vi "Process.vi"(8 "error in":errorcluster, 11 "Instrument.AFM_DLog in":refnum<class "Instrument.AFM_DLog.lvclass">) -> (0 "error out":errorcluster, 3 "Instrument.AFM_DLog out":refnum<class "Instrument.AFM_DLog.lvclass">)   [LabVIEW 2019, in "Instrument.AFM_DLog.lvclass"]
doc: "---------------------------------------------------------------\nJKI State Machine Objects™\nhttp://jki.net/state-machine-objects/\nCopyright (C) 2005-2015, JKI <info@jki.net>\nALL RIGHTS RESERVED"
uses:
  Instrument.AFM_DLog.lvclass
  <vilib>/JKI/JKI SMO/SMO/SMO.lvclass
  <userlib>/LevyLab/Instrument Framework/Instrument/Instrument.lvclass
  <userlib>/LevyLab/RemoteControl/RemoteControl/Typedefs/Message--Cluster.ctl
  <userlib>/LevyLab/RemoteControl/RemoteControl/RemoteControl.lvclass
  Typedefs/PrivateEvents--AFM_DLog.MessageToProcess.ctl
  <userlib>/LevyLab/Instrument Framework/Instrument Types/SCPI/Instrument.SCPI.lvclass
  <userlib>/LevyLab/Debug/Debug.lvlib
  <userlib>/LevyLab/Instrument Framework/Instrument/API/Instrument.sendMessageToProcess (string).vi
  C:/Program Files (x86)/National Instruments/LabVIEW 2019/vi.lib/JKI/JKI SMO/SMO/SMO.lvclass
  C:/Program Files (x86)/National Instruments/LabVIEW 2019/user.lib/LevyLab/Instrument Framework/Instrument/Instrument.lvclass
panel:
  out "Status":string
  out "State History":string
  # "Instrument.Framework-Template"
  # "Framework-Template"
  # "For instructions on how to use the JKI State Machine Objects, examples and video tutorials, visit:\nhttp://jki.net/state-machine-objects/\n\nJKI State Machine Objects™\nhttp://jki.net/state-machine-objects/\nCopyright (C) 2005-2015, JKI <info@jki.net>\nALL RIGHTS RESERVED"
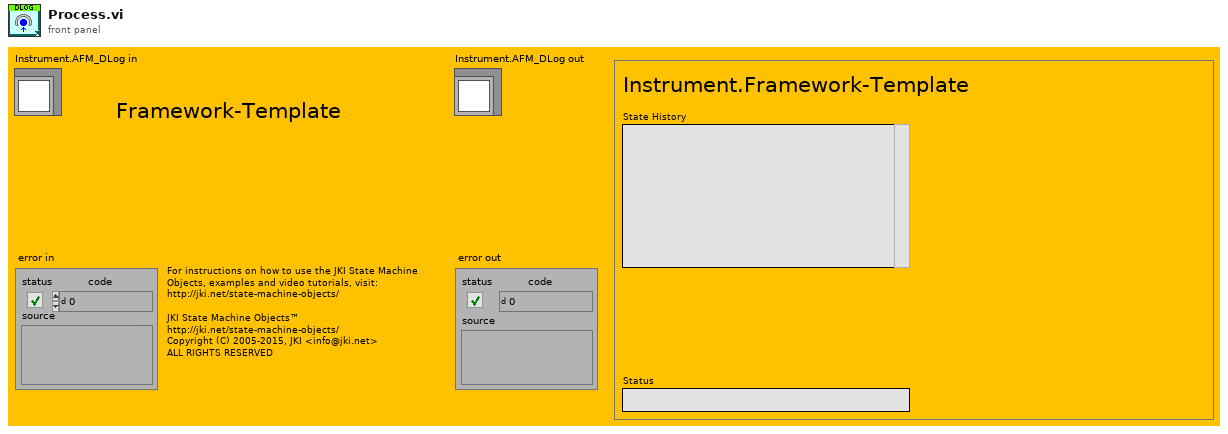
[diagram p1: front panel]
types:
  T1 = enum32{"invalid app kind", "Development System", "Run Time System", "Student Edition", "Embedded LabVIEW", "Evaluation", "Custom"}
  T2 = enum32{"Invalid", "Standard", "Closed", "Hidden", "Minimized", "Maximized"}
  T3 = typedef "RemoteControl.lvlib/RemoteControl.lvclass/Message--Cluster.ctl" = cluster{"Command":string, "Data":variant, "ID":string}
  T4 = typedef "Instrument.AFM_DLog.lvclass/PrivateEvents--AFM_DLog.MessageToProcess.ctl" = cluster{"Message":T3}
  T5 = cluster{"Core":cluster{"Current VI Reference":refnum<vi>, "Close Panel on Exit?":bool, "Last Error":cluster{"error":errorcluster, "previous state":string, "remaining states":string}, "Shutdown?":bool}, "SelfRef":refnum<class "Instrument.AFM_DLog.lvclass">, "HAL":refnum<class "HAL.lvclass">, "Running Step":i32, "sequence":string[], "MessageToProcess":T4, "UI Behavior":string, "wait":u32}
  T6 = cluster{"Current VI Reference":refnum<vi>, "Close Panel on Exit?":bool, "Last Error":cluster{"error":errorcluster, "previous state":string, "remaining states":string}, "Shutdown?":bool}
  T7 = typedef "Debug.lvlib/Attribute.Debug.lvclass/DebugBehavior.ctl" = enum16{"Normal", "Debug"}
  T8 = typedef "smo.lvlib/SMO.lvclass/Protected Events.ctl" = cluster{"StopProcesses":refnum<user-event>, "AbortProcesses":refnum<user-event>, "Config Changed":refnum<user-event>, "Dependency":refnum<user-event>}
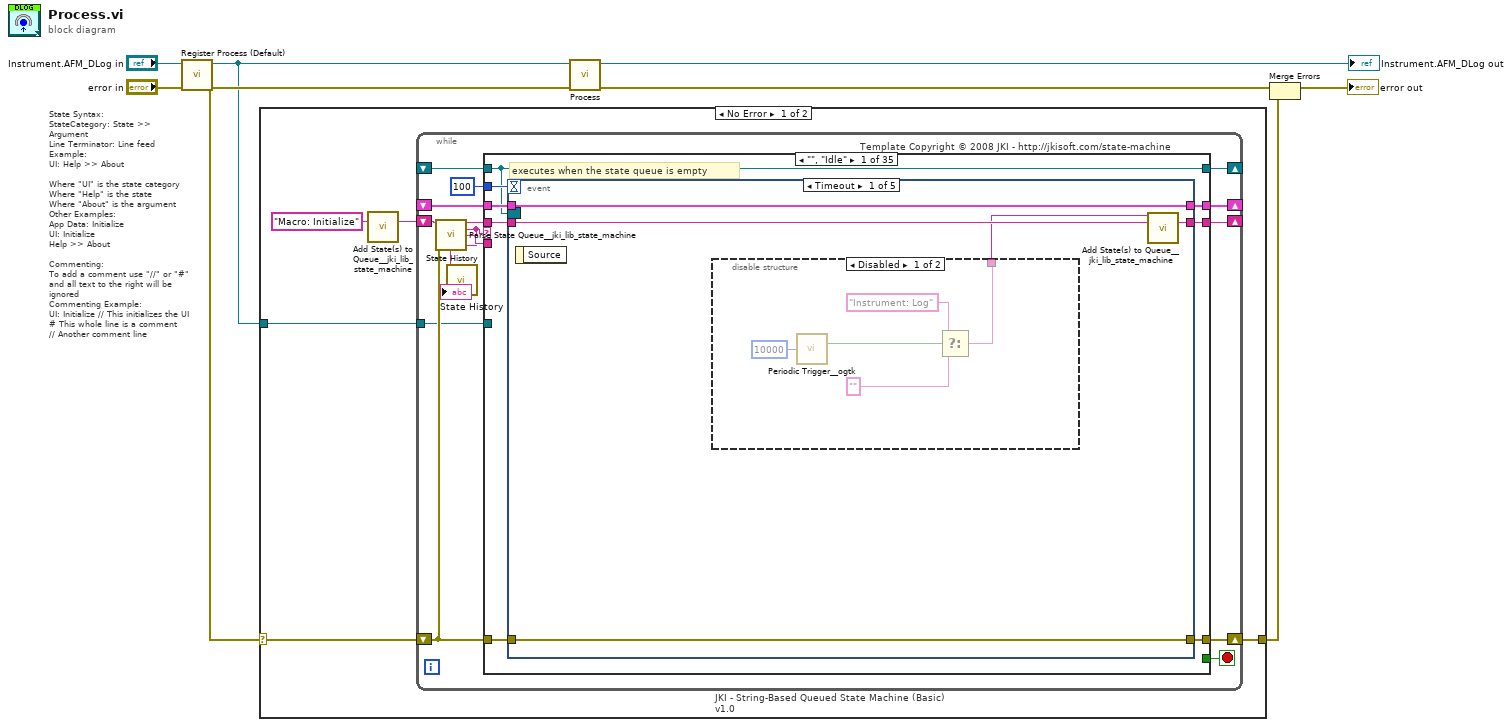
[diagram p0: block diagram]
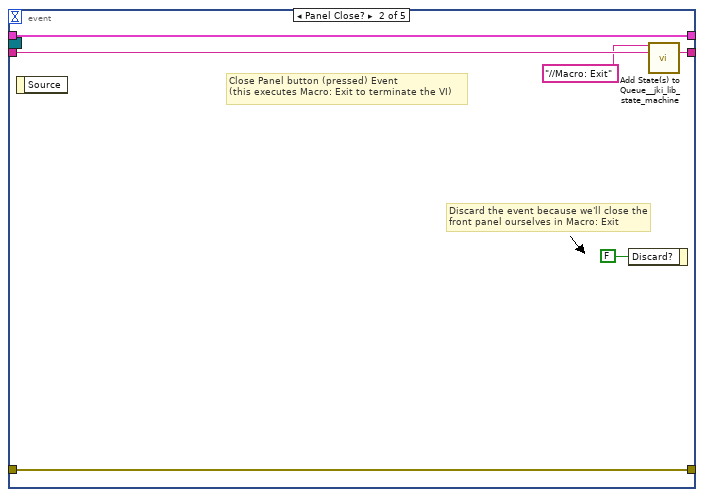
[diagram p3: hidden frame]
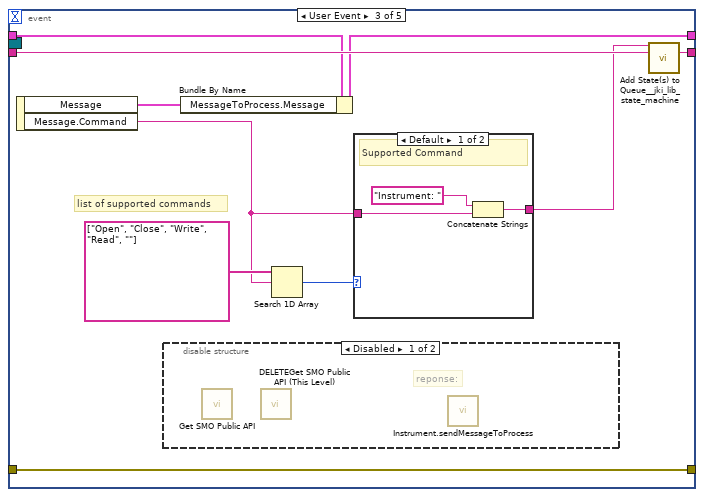
[diagram p4: hidden frame]
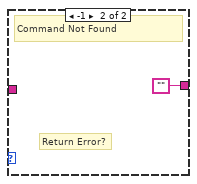
[diagram p6: hidden frame]
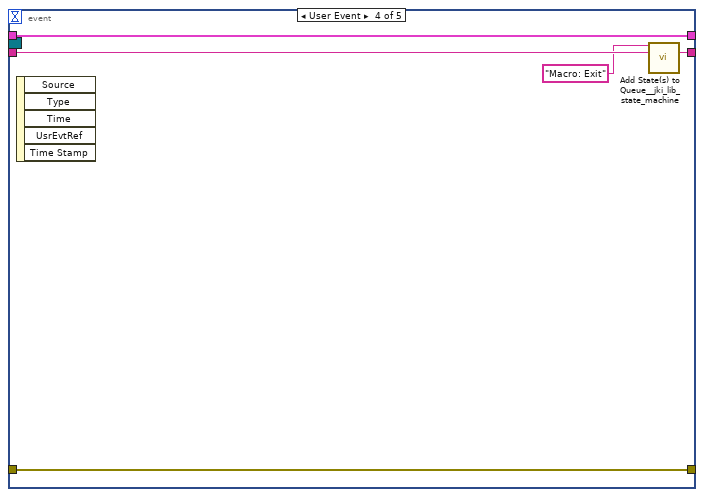
[diagram p7: hidden frame]
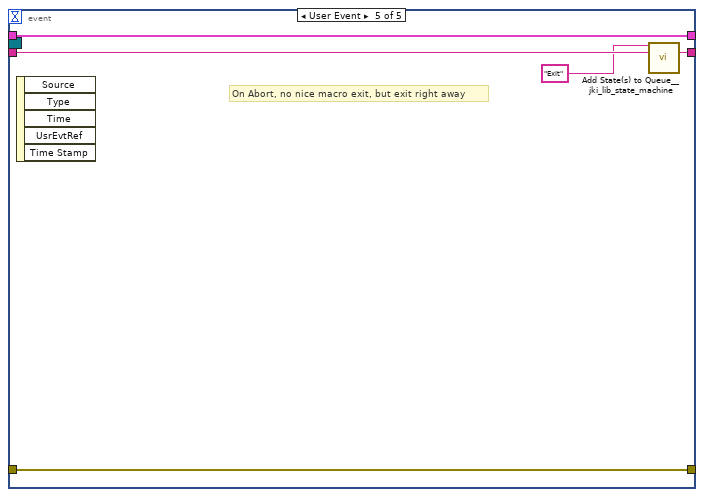
[diagram p8: hidden frame]
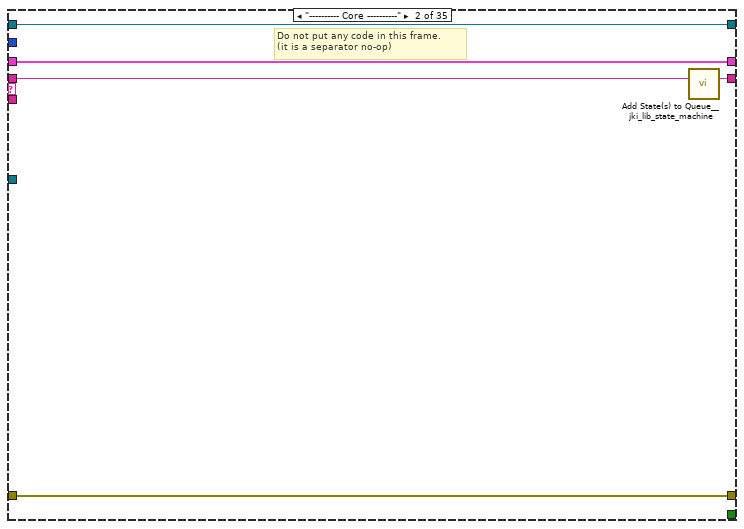
[diagram p9: hidden frame]
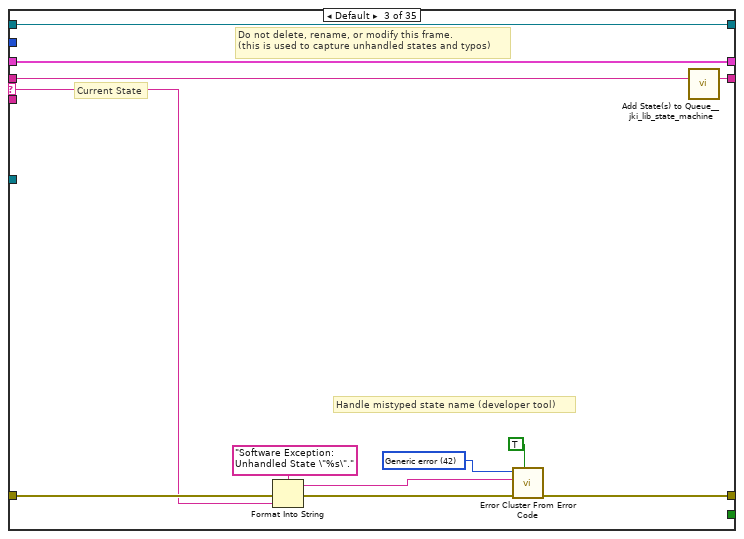
[diagram p10: hidden frame]
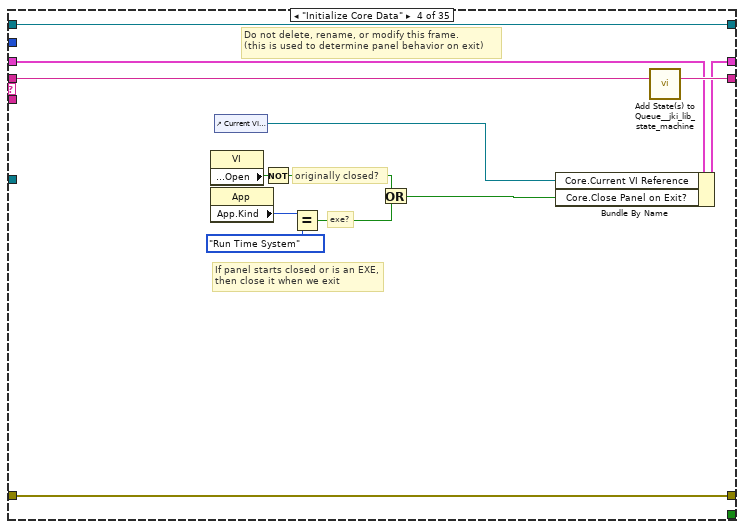
[diagram p11: hidden frame]
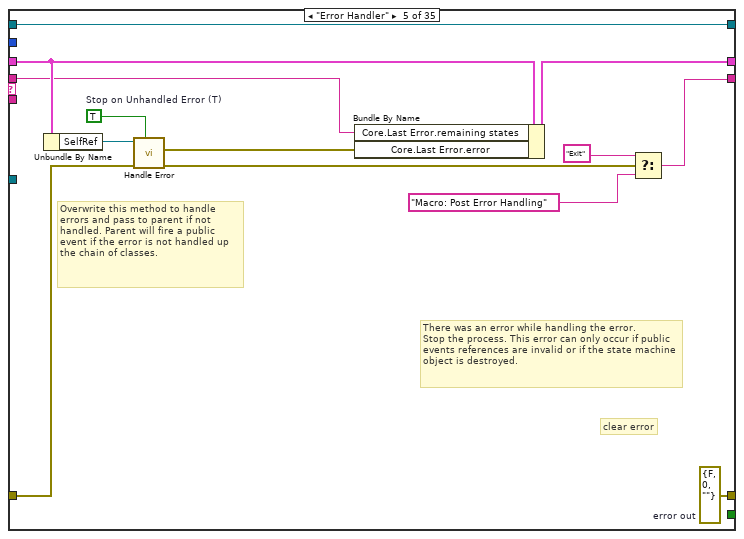
[diagram p12: hidden frame]
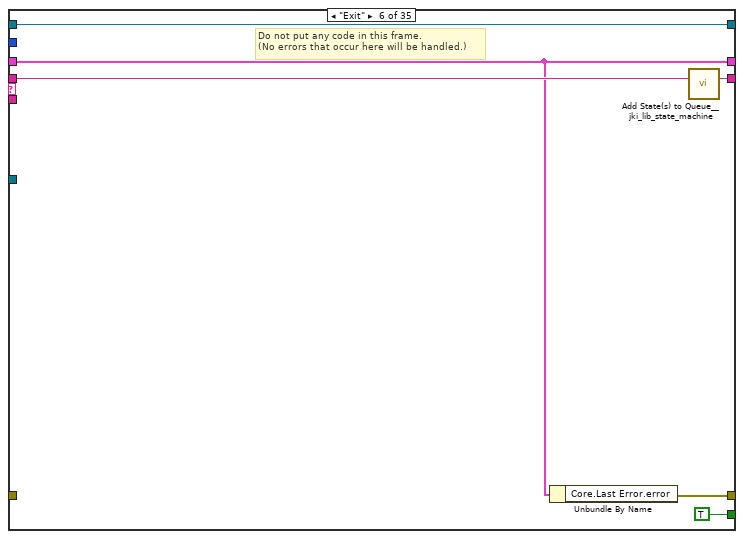
[diagram p13: hidden frame]
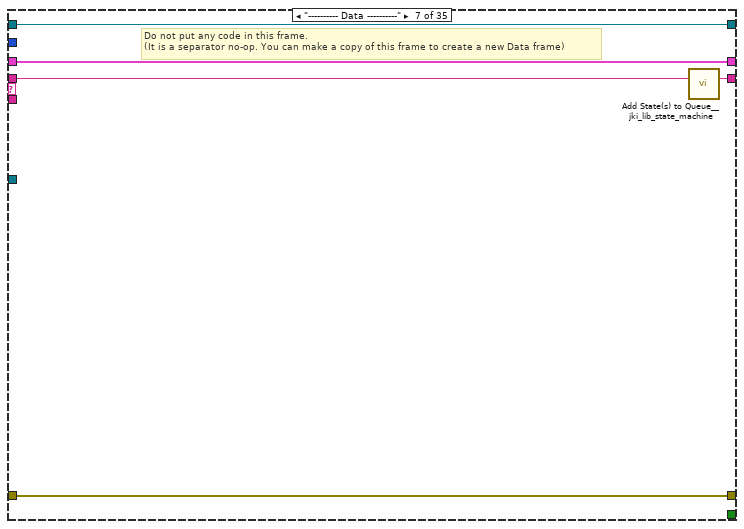
[diagram p14: hidden frame]
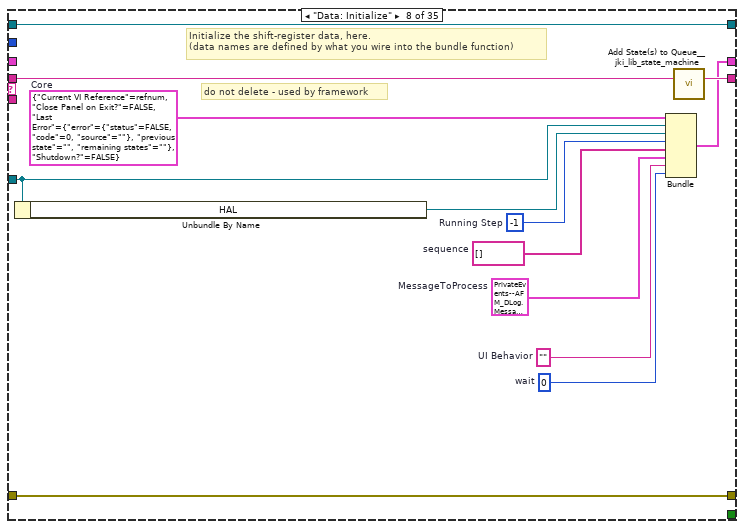
[diagram p15: hidden frame]
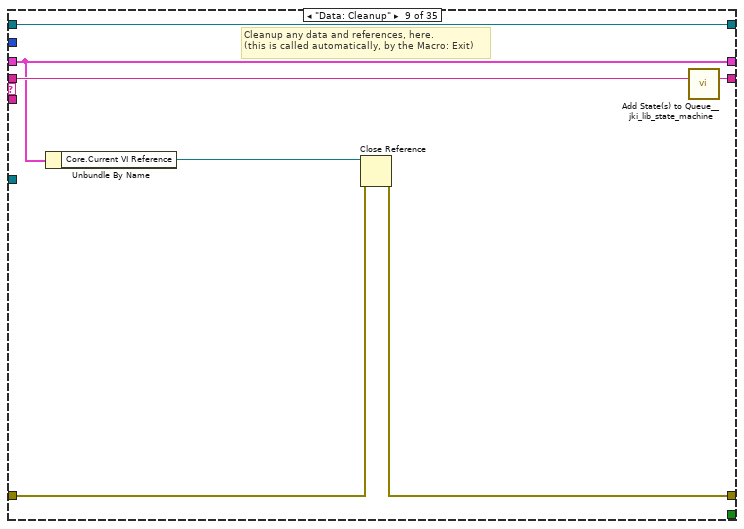
[diagram p16: hidden frame]
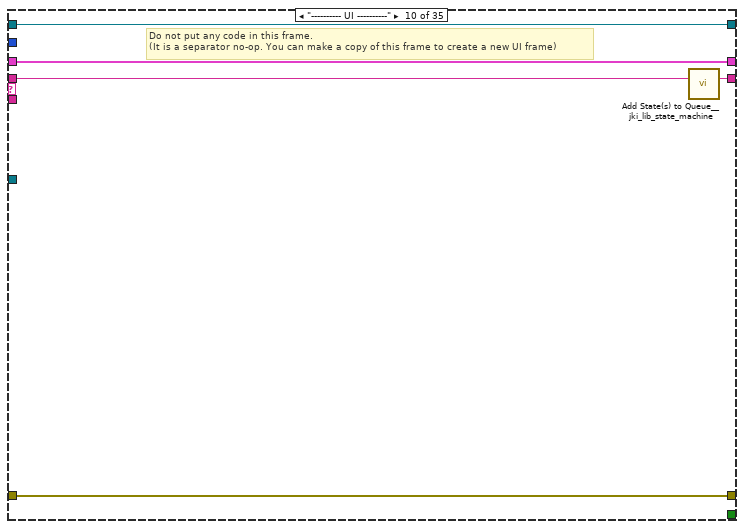
[diagram p17: hidden frame]
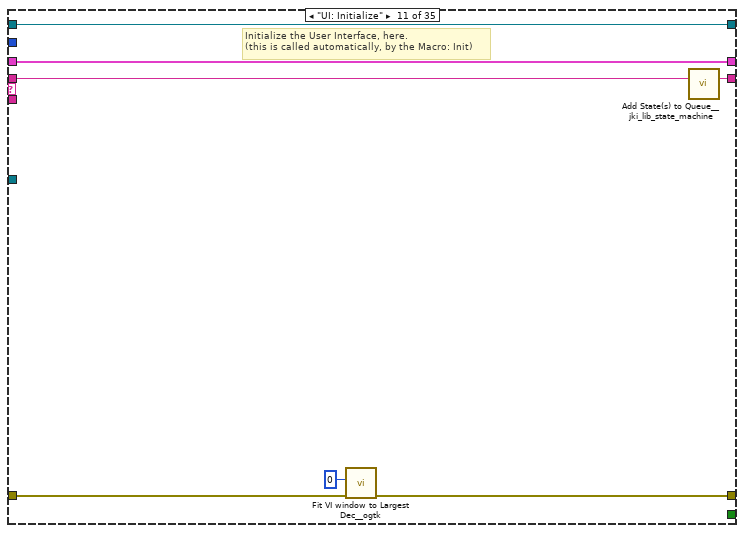
[diagram p18: hidden frame]
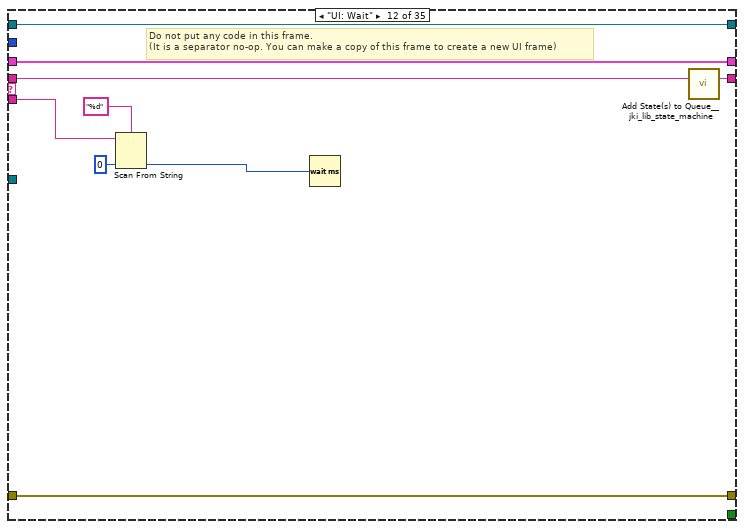
[diagram p19: hidden frame]
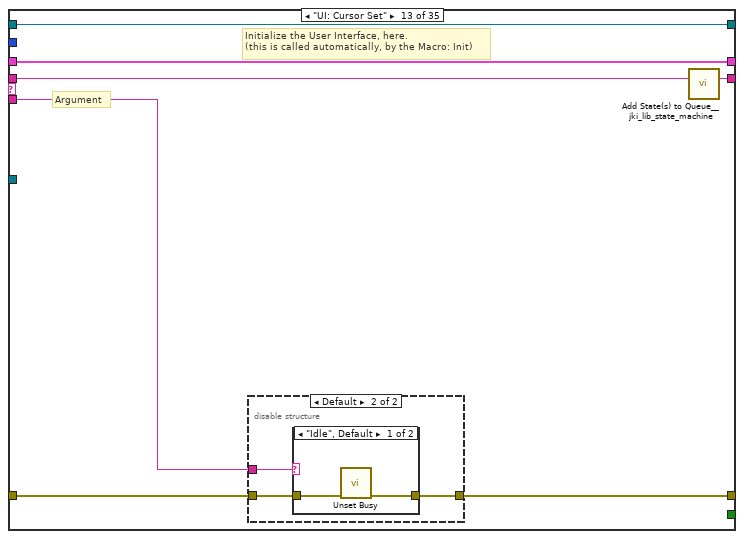
[diagram p20: hidden frame]
diagram:
  # "State Syntax:\nStateCategory: State >> Argument\nLine Terminator: Line feed\nExample:\nUI: Help >> About\n\nWhere \"UI\" is the state category\nWhere \"Help\" is the state\nWhere \"About\" is the argument\nOther Examples:\nApp Data: Initialize\nUI: Initialize\nHelp >> About\n\nCommenting:\nTo add a comment use \"//\" or \"#\" and all text to the right will be ignored\nCommenting Example:\nUI: Initialize // This initializes the UI\n# This whole line is a comment\n// Another comment line"
  n1 = call <vilib>:"Register Process (Default).vi"("error in (no error)"="error in", "SMO"="Instrument.AFM_DLog in") -> ("error out"=w5:errorcluster, "SelfRef"=w4:refnum<class "Instrument.AFM_DLog.lvclass">)  [unwired: 8 in]
  n2 = case shown="No Error" w5 {
    selector: w5 -> [w10 w455]
    tunnel: w4 -> [w11 _]
    tunnel: [w9 w455] -> w1
    frame No Error {
      n3 = call <vilib>:"Add State(s) to Queue__jki_lib_state_machine.vi"("State(s) in (\"\")"="Macro: Initialize") -> ("States Out"=w13:string)  [unwired: 14 in]
      n4 = while "JKI - String-Based Queued State Machine (Basic) v1.0" {
        shift-right: [w22] -> _
        shift-left: _ -> [w21]
        shift-right: [w25] -> w9
        shift-left: w10 -> [w19]
        shift-right: [w24] -> _
        shift-left: w13 -> [w26]
        tunnel: w11 -> [w18]
        shift-right: [w17] -> _
        shift-left: _ -> [w16]
        stop <- w23 stop-if-true
        # "Template Copyright © 2008 JKI - http://jkisoft.com/state-machine"
        n5 = call <vilib>:"Parse State Queue__jki_lib_state_machine.vi"("State Queue"=w26, "Error In (no error)"=w19) -> ("Remaining States"=w28:string, "Current State"=w15:string, "Arguments"=w27:string)  [unwired: 11 in]
        n6 = call <userlib>:"State History.vi"("Current State"=w15) -> ("History"=→"State History":string)  [unwired: 10 in]
        n7 = case shown="\"\", \"Idle\"" w15 {
          selector: w15 -> [_ _ w83 _ _ _ _ _ _ _ _ _ _ _ _ _ _ _ _ _ _ _ _ _ _ _ _ _ _ _ _ _ _ _ _]
          tunnel: w28 -> [w36 w81 w87 w106 w111 w125 w130 w143 w150 w155 w162 w171 w178 w194 w226 w235 w247 w268 w283 w305 w310 w321 w326 w339 w345 w353 w362 w371 w381 w390 w405 w424 w429 w435 w454]
          tunnel: w27 -> [_ _ _ _ _ _ _ _ _ _ _ w163 w172 w188 _ _ _ _ _ _ _ _ _ _ _ _ _ _ _ _ _ _ _ w430 w438]
          tunnel: w21 -> [w34 w78 w85 w97 w115 w121 w127 _ w145 w152 w160 w168 w176 w190 w223 w232 w237 w258 w272 w290 w307 w318 w323 w332 w343 w348 w358 w367 w377 w386 w401 w420 w425 w431 w444]
          tunnel: [w33 w79 w89 w103 w116 w120 w128 w133 w146 w153 w157 w169 w173 w191 w224 w227 w245 w266 w271 w293 w308 w312 w324 w335 w341 w350 w354 w366 w376 w385 w395 w418 w426 w432 w446] -> w25
          tunnel: w19 -> [w32 w79 w88 w103 w117 _ w128 w133 w147 w153 w156 w169 w174 w192 w224 w227 w245 w266 w270 w293 w308 w313 w324 w329 w341 w350 w357 w365 w375 w384 w399 w416 w426 w432 w440]
          tunnel: [w35 w80 w86 w105 w107 w124 w129 w142 w149 w154 w161 w170 w177 w193 w225 w234 w246 w267 w282 w304 w309 w320 w325 w338 w344 w352 w361 w370 w380 w389 w404 w423 w428 w434 w453] -> w24
          tunnel: [_ _ _ _ _ TRUE _ _ _ _ _ _ _ _ _ _ _ _ _ _ _ _ _ _ _ _ _ _ _ _ _ _ _ _ _] -> w23
          tunnel: [w31 w78 w85 w104 w114 w121 w127 w141 w145 w152 w160 w168 w176 w190 w223 w232 w238 w259 w273 w291 w307 w318 w323 w332 w343 w349 w359 w368 w378 w387 w402 w421 w425 w431 w443] -> w22
          tunnel: 100 ("Timeout") -> [w30 _ _ _ _ _ _ _ _ _ _ _ _ _ _ _ _ _ _ _ _ _ _ _ _ _ _ _ _ _ _ _ _ _ _]
          tunnel: w18 -> [_ _ _ _ _ _ _ w134 _ _ _ _ _ _ _ _ _ _ _ _ _ _ _ _ _ _ _ _ _ _ _ _ _ _ _]
          tunnel: [w29 w77 w82 w94 w119 w122 w126 w140 w144 w151 w159 w167 w175 w187 w222 w233 w244 w265 w281 w299 w306 w319 w322 w337 w342 w351 w360 w369 w379 w388 w403 w422 w427 w433 w452] -> w17
          tunnel: w16 -> [w29 w77 w82 w94 w119 w122 w126 w140 w144 w151 w159 w167 w175 w187 w222 w233 w244 w265 w281 w299 w306 w319 w322 _ w342 w351 w360 w369 w379 w388 w403 w422 w427 w433 w452]
          frame "", "Idle" {
            # "executes when the state queue is empty"
            n8 = event shown="[0] Timeout" {
              selector: w29 -> [_ _ _ _ _]
              dyn-events: _ -> [_ _ _ _ _]
              timeout: w30 -> [_ _ _ _ _]
              tunnel: w36 -> [w41 w52 w62 w71 w76]
              tunnel: [w40 w51 w61 w70 w75] -> w35
              tunnel: w34 -> [w38 w49 w54 w68 w73]
              tunnel: [w39 w50 w60 w69 w74] -> w33
              tunnel: w32 -> [w39 w50 w60 w69 w74]
              tunnel: [w38 w49 w55 w68 w73] -> w31
              event Timeout {
                n9 = event-data() -> ()  [unwired: 1 in, 1 out]
                n10 = disable-structure shown="Disabled" {
                  disable-tunnel: [w45 _] -> w37
                  frame Disabled {
                    n11 = call <userlib>:"Periodic Trigger__ogtk.vi"("time (ms)"=u32 10000) -> ("Triggered"=w44:bool)  [unwired: 12 in, 2 out]
                    n12 = Select(t="Instrument: Log", s=w44, f="") -> (s? t:f=w45:string)
                  }
                  frame Enabled {
                  }
                }
                n13 = call <vilib>:"Add State(s) to Queue__jki_lib_state_machine.vi"("State(s) in Front (\"\")"=w37, "State(s) in (\"\")"=w41) -> ("States Out"=w40:string)  [unwired: 13 in]
              }
              event Panel Close? {
                # "Discard the event because we'll close the front panel ourselves in Macro: Exit"
                # "Close Panel button (pressed) Event\n(this executes Macro: Exit to terminate the VI)"
                n14 = event-data() -> ()  [unwired: 1 in, 1 out]
                n15 = event-data("Discard?"=FALSE) -> ()  [unwired: 1 in, 1 out]
                n16 = call <vilib>:"Add State(s) to Queue__jki_lib_state_machine.vi"("State(s) in Front (\"\")"="//Macro: Exit", "State(s) in (\"\")"=w52) -> ("States Out"=w51:string)  [unwired: 13 in]
              }
              event User Event {
                # "list of supported commands"
                n17 = event-data() -> ("Message"=w53:T3, "Message.Command"=w56:string)  [unwired: 1 in]
                n18 = disable-structure shown="Disabled" {
                  frame Disabled {
                    # "reponse:"
                    n19 = call-dynamic "Get SMO Public API.vi"() -> ()  [unwired: 9 in, 3 out]
                    n20 = call-dynamic "DELETEGet SMO Public API (This Level).vi"() -> ()  [unwired: 9 in, 3 out]
                    n21 = call-poly <userlib>:"Instrument.sendMessageToProcess.vi"() -> ()  [unwired: 10 in, 2 out]
                  }
                  frame Enabled {
                  }
                }
                n22 = Bundle By Name(cluster=w54, "MessageToProcess.Message"=w53) -> (w55:T5)
                n23 = Search 1D Array(1D array=string[] ["Open", "Close", "Write", "Read", ""], element=w56) -> (index of element=w59:i32)  [unwired: 1 in]
                n24 = case shown="Default" w59 {
                  tunnel: [w65 "" ("Empty String Constant")] -> w57
                  tunnel: w56 -> [w64 _]
                  frame Default {
                    # "Supported Command"
                    n25 = Concatenate Strings("Instrument: ", w64) -> (w65:string)
                  }
                  frame -1 {
                    # "Return Error?"
                    # "Command Not Found"
                  }
                }
                n26 = call <vilib>:"Add State(s) to Queue__jki_lib_state_machine.vi"("State(s) in Front (\"\")"=w57, "State(s) in (\"\")"=w62) -> ("States Out"=w61:string)  [unwired: 13 in]
              }
              event User Event {
                n27 = event-data() -> ()  [unwired: 1 in, 5 out]
                n28 = call <vilib>:"Add State(s) to Queue__jki_lib_state_machine.vi"("State(s) in Front (\"\")"="Macro: Exit", "State(s) in (\"\")"=w71) -> ("States Out"=w70:string)  [unwired: 13 in]
              }
              event User Event {
                # "On Abort, no nice macro exit, but exit right away"
                n29 = event-data() -> ()  [unwired: 1 in, 5 out]
                n30 = call <vilib>:"Add State(s) to Queue__jki_lib_state_machine.vi"("State(s) in Front (\"\")"="Exit", "State(s) in (\"\")"=w76) -> ("States Out"=w75:string)  [unwired: 13 in]
              }
            }
          }
          frame "---------- Core ----------" {
            # "Do not put any code in this frame.\n(it is a separator no-op)"
            n31 = call <vilib>:"Add State(s) to Queue__jki_lib_state_machine.vi"("State(s) in (\"\")"=w81) -> ("States Out"=w80:string)  [unwired: 14 in]
          }
          frame Default {
            w92 = 42 items=["No error", "Argument error", "Memory is full", "Out of zone", "End of file", "File already open", "Generic file I/O error", "File not found", "File permission error", "Disk is full", "Duplicate path", "Too many files open", "System feature not enabled", "Resource file not found", "Cannot add resource", "Resource not found", "Image not found", "Image memory error", "Pen does not exist", "Config type invalid", "Config token not found", "Config parse error", "Config memory error", "Bad external code format", "Bad external code offset", "External code not present", "Null window", "Destroy window error", "Null menu", "Print aborted", "Bad print record", "Print driver error", "Windows error during printing", "Memory error during printing", "Print dialog error", "Generic print error", "Invalid device refnum", "Device not found", "Device parameter error", "Device unit error", "Cannot open device", "Device call aborted", "Generic error", "Cancelled by user", "Object ID too low", "Object ID too high", "Object not in heap", "Unknown heap", "Unknown object (invalid DefProc)", "Unknown object (DefProc not in table)", "Message out of range", "Invalid (null) method", "Unknown message", "Manager call not supported", "Bad address", "Network operation in progress", "Network operation timed out", "Connection is busy", "Network attribute not supported", "Network error", "Address in use", "System out of memory", "Connection aborted", "Connection refused", "Not connected", "Already connected", "Connection closed", "Initialization error (interapplication manager)", "Bad occurrence", "Wait on unbound occurrence handler", "Occurrence queue overflow", "Datalog type conflict", "Unused", "Unrecognized type (interapplication manager)", "Memory corrupt", "Failed to make temporary DLL", "Old CIN version", "Drag socket not found", "Failed to load drop-object", "Failed to register OLE object", "Failed to release OLE object", "Format specifier type mismatch", "Unknown format specifier", "Too few format specifiers", "Too many format specifiers", "Scan failed", "Newer CIN version", "Error converting to variant", "Runtime menu error", "Password tampered", "Variant attribute not found", "Incompatible variant data type", "Event data is not available", "Event Store is not present", "Occurrence is not found", "Event Queue is not created", "Event info is not available", "Refnum passed is NULL", "Error retrieving Class GUID", "Error retrieving CoClass GUID", "Error retrieving TypeLib GUID.", "Bad built application magic bytes.", "Specific driver is different from the specific driver associated with the Logical Name.", "There is no session opened to the class driver.", "Max Error", "MAX - Error with config objects", "MAX - Error loading configuration", "MAX - Group not supported"]
            # "Current State"
            # "Do not delete, rename, or modify this frame.\n(this is used to capture unhandled states and typos)"
            # "Handle mistyped state name (developer tool)"
            n32 = Format Into String(format string="Software Exception: Unhandled State \"%s\"." ("message"), error in=w88, w83) -> (resulting string=w91:string, error out=w90:errorcluster)  [unwired: 1 in]
            n33 = call <vilib>:"Error Cluster From Error Code.vi"("show call chain? (False)"=TRUE, "error in (no error)"=w90, "error message (\"\")"=w91, "error code (0)"=w92) -> ("error out"=w89:errorcluster)  [unwired: 5 in]
            n34 = call <vilib>:"Add State(s) to Queue__jki_lib_state_machine.vi"("State(s) in (\"\")"=w87) -> ("States Out"=w86:string)  [unwired: 14 in]
          }
          frame "Initialize Core Data" {
            # "Do not delete, rename, or modify this frame.\n(this is used to determine panel behavior on exit)"
            # "originally closed?"
            # "exe?"
            # "If panel starts closed or is an EXE, then close it when we exit"
            n35 = property class="VI"() -> ("Front Panel.Open"=w102:bool)  [unwired: 2 in, 2 out]
            n36 = property class="App"() -> ("App.Kind"=w101:T1)  [unwired: 2 in, 2 out]
            n37 = control-ref of="Current VI Reference"() -> (w95:refnum<vi>)
            n38 = Not(x=w102) -> (.not. x?=w99:bool)
            n39 = Equal?(x=w101, y=T1."Run Time System" ("Application:Kind")) -> (x = y?=w98:bool)
            n40 = Or(x=w99, y=w98) -> (x .or. y?=w96:bool)
            n41 = Bundle By Name(cluster=w97, "Core.Current VI Reference"=w95, "Core.Close Panel on Exit?"=w96) -> (w104:T5)
            n42 = call <vilib>:"Add State(s) to Queue__jki_lib_state_machine.vi"("State(s) in (\"\")"=w106) -> ("States Out"=w105:string)  [unwired: 14 in]
          }
          frame "Error Handler" {
            w112 = TRUE  # Stop on Unhandled Error (T)
            w116 = errorcluster {"status"=FALSE, "code"=0, "source"=""}  # error out
            # "clear error"
            # "There was an error while handling the error.\nStop the process. This error can only occur if public events references are invalid or if the state machine object is destroyed."
            # "Overwrite this method to handle errors and pass to parent if not handled. Parent will fire a public event if the error is not handled up the chain of classes."
            n43 = Unbundle By Name(w115) -> ("SelfRef"=w118:refnum<class "Instrument.AFM_DLog.lvclass">)
            n44 = call-dynamic "Handle Error.vi"("Stop on Unhandled Error (T)"=w112, "error in"=w117, "SMO"=w118) -> ("handling error"=w108:errorcluster, "Unhandled error"=w113:errorcluster)  [unwired: 6 in, 1 out]
            n45 = Bundle By Name(cluster=w115, "Core.Last Error.remaining states"=w111, "Core.Last Error.error"=w113) -> (w114:T5)
            n46 = Select(t="Exit", s=w108, f="Macro: Post Error Handling") -> (s? t:f=w107:string)
          }
          frame "Exit" {
            # "Do not put any code in this frame.\n(No errors that occur here will be handled.)"
            n47 = Unbundle By Name(w121) -> ("Core.Last Error.error"=w120:errorcluster)
            n48 = call <vilib>:"Add State(s) to Queue__jki_lib_state_machine.vi"("State(s) in (\"\")"=w125) -> ("States Out"=w124:string)  [unwired: 14 in]
          }
          frame "---------- Data ----------" {
            # "Do not put any code in this frame.\n(It is a separator no-op. You can make a copy of this frame to create a new Data frame)"
            n49 = call <vilib>:"Add State(s) to Queue__jki_lib_state_machine.vi"("State(s) in (\"\")"=w130) -> ("States Out"=w129:string)  [unwired: 14 in]
          }
          frame "Data: Initialize" {
            w131 = u32 0  # wait
            w132 = ""  # UI Behavior
            w136 = T4 {"Message"={"Command"="", "Data"=variant(string ""), "ID"=""}}  # MessageToProcess
            w137 = string[] []  # sequence
            w138 = -1  # Running Step
            w139 = T6 {"Current VI Reference"=refnum, "Close Panel on Exit?"=FALSE, "Last Error"={"error"={"status"=FALSE, "code"=0, "source"=""}, "previous state"="", "remaining states"=""}, "Shutdown?"=FALSE}  # Core
            # "do not delete - used by framework"
            # "Initialize the shift-register data, here.\n(data names are defined by what you wire into the bundle function)"
            n50 = Unbundle By Name(w134) -> ("HAL"=w135:refnum<class "HAL.lvclass">)
            n51 = Bundle("Core"=w139, "SelfRef"=w134, "HAL"=w135, "Running Step"=w138, "sequence"=w137, "MessageToProcess"=w136, "UI Behavior"=w132, "wait"=w131) -> (w141:T5)  [unwired: 1 in]
            n52 = call <vilib>:"Add State(s) to Queue__jki_lib_state_machine.vi"("State(s) in (\"\")"=w143) -> ("States Out"=w142:string)  [unwired: 14 in]
          }
          frame "Data: Cleanup" {
            # "Cleanup any data and references, here.\n(this is called automatically, by the Macro: Exit)"
            n53 = Unbundle By Name(w145) -> ("Core.Current VI Reference"=w148:refnum<vi>)
            n54 = Close Reference(reference=w148, error in (no error)=w147) -> (error out=w146:errorcluster)
            n55 = call <vilib>:"Add State(s) to Queue__jki_lib_state_machine.vi"("State(s) in (\"\")"=w150) -> ("States Out"=w149:string)  [unwired: 14 in]
          }
          frame "---------- UI ----------" {
            # "Do not put any code in this frame.\n(It is a separator no-op. You can make a copy of this frame to create a new UI frame)"
            n56 = call <vilib>:"Add State(s) to Queue__jki_lib_state_machine.vi"("State(s) in (\"\")"=w155) -> ("States Out"=w154:string)  [unwired: 14 in]
          }
          frame "UI: Initialize" {
            # "Initialize the User Interface, here.\n(this is called automatically, by the Macro: Init)"
            n57 = call <userlib>:"Fit VI window to Largest Dec__ogtk.vi"("error in (no error)"=w156, "border spacing (2 px)"=0) -> ("error out"=w157:errorcluster)  [unwired: 4 in, 1 out]
            n58 = call <vilib>:"Add State(s) to Queue__jki_lib_state_machine.vi"("State(s) in (\"\")"=w162) -> ("States Out"=w161:string)  [unwired: 14 in]
          }
          frame "UI: Wait" {
            # "Do not put any code in this frame.\n(It is a separator no-op. You can make a copy of this frame to create a new UI frame)"
            n59 = Scan From String(format string="%d", input string=w163, default 1=u32 0 ("default value 1")) -> (output 1=w164:u32)  [unwired: 2 in, 3 out]
            n60 = Wait (ms)(milliseconds to wait=w164) -> ()  [unwired: 1 out]
            n61 = call <vilib>:"Add State(s) to Queue__jki_lib_state_machine.vi"("State(s) in (\"\")"=w171) -> ("States Out"=w170:string)  [unwired: 14 in]
          }
          frame "UI: Cursor Set" {
            # "Argument"
            # "Initialize the User Interface, here.\n(this is called automatically, by the Macro: Init)"
            n62 = disable-structure shown="Default" {
              disable-tunnel: w174 -> [w179 w182]
              disable-tunnel: [w179 w181] -> w173
              disable-tunnel: w172 -> [_ w180]
              frame condition #0 {
              }
              frame condition #1 (active) {
                n63 = case shown="\"Idle\", Default" w180 {
                  tunnel: w182 -> [w184 w186]
                  tunnel: [w183 w185] -> w181
                  frame "Idle", Default {
                    n64 = call <vilib>:"Unset Busy.vi"("error in (no error)"=w184) -> ("error out"=w183:errorcluster)  [unwired: 10 in]
                  }
                  frame "Busy" {
                    n65 = call <vilib>:"Set Busy.vi"("error in (no error)"=w186) -> ("error out"=w185:errorcluster)  [unwired: 9 in, 1 out]
                  }
                }
              }
            }
            n66 = call <vilib>:"Add State(s) to Queue__jki_lib_state_machine.vi"("State(s) in (\"\")"=w178) -> ("States Out"=w177:string)  [unwired: 14 in]
          }
          frame "UI: Front Panel State" {
            # "Argument"
            # "Set Front Panel Open or Closed\n(Usage: \"UI: Front Panel State >> Open|Close\")"
            n67 = Unbundle By Name(w190) -> ("Core.Current VI Reference"=w189:refnum<vi>)
            n68 = disable-structure shown="TARGET_TYPE==RT" {
              disable-tunnel: w192 -> [w198 w221]
              disable-tunnel: [w197 w221] -> w191
              disable-tunnel: w189 -> [w196 _]
              disable-tunnel: w188 -> [w195 _]
              frame condition #0 (active) {
                n69 = case shown="\"Close\"" w195 {
                  tunnel: w198 -> [w202 w215]
                  tunnel: [w204 w216] -> w197
                  tunnel: w196 -> [w203 w213]
                  frame "Open", Default {
                    n70 = property class="VI"(reference=w203, error in=w202) -> (reference out=w200:refnum<vi>, error out=w201:errorcluster, "FP.State"=w199:T2)
                    n71 = case shown="\"Closed\"" w199 {
                      tunnel: [w207 w210] -> w204
                      tunnel: w201 -> [w206 w210]
                      tunnel: w200 -> [w205 _]
                      frame "Closed" {
                        n72 = invoke class="VI" method="FP.Open"(reference=w205, error in=w206, "Activate"=TRUE, "State"=T2."Standard") -> (error out=w207:errorcluster)  [unwired: 1 in, 4 out]
                      }
                      frame Default {
                      }
                    }
                  }
                  frame "Close" {
                    n73 = property class="VI"(reference=w213, error in=w215) -> (reference out=w212:refnum<vi>, error out=w214:errorcluster, "FP.State"=w211:T2)
                    n74 = case shown="Default" w211 {
                      tunnel: [w217 w220] -> w216
                      tunnel: w214 -> [w217 w219]
                      tunnel: w212 -> [_ w218]
                      frame "Invalid", "Closed" {
                      }
                      frame Default {
                        n75 = invoke class="VI" method="FP.Close"(reference=w218, error in=w219) -> (error out=w220:errorcluster)  [unwired: 1 in, 2 out]
                      }
                    }
                  }
                }
              }
              frame condition #1 {
              }
            }
            n76 = call <vilib>:"Add State(s) to Queue__jki_lib_state_machine.vi"("State(s) in (\"\")"=w194) -> ("States Out"=w193:string)  [unwired: 14 in]
          }
          frame "---------- Macro ----------" {
            # "Do not put any code in this frame.\n(It is a separator no-op. You can make a copy of this frame to create a new Macro frame)"
            n77 = call <vilib>:"Add State(s) to Queue__jki_lib_state_machine.vi"("State(s) in (\"\")"=w226) -> ("States Out"=w225:string)  [unwired: 14 in]
          }
          frame "Macro: Initialize" {
            # "Initialization Macro\n(This is called once, when the VI starts)"
            n78 = call <vilib>:"Add State(s) to Queue__jki_lib_state_machine.vi"("State(s) in Front (\"\")"="Data: Initialize\nInitialize Core Data\nEvents: Register", "State(s) in (\"\")"="Process: Sync", "State(s) at Back (\"\")"="UI: Initialize\nUI: Front Panel State >> Close\nInstrument: Open\nMacro: Debug") -> ("States Out"=w230:string)  [unwired: 12 in]
            n79 = call <vilib>:"Add State(s) to Queue__jki_lib_state_machine.vi"("State(s) in Front (\"\")"=w230, "State(s) in (\"\")"=w235) -> ("States Out"=w234:string)  [unwired: 13 in]
          }
          frame "Macro: Post Error Handling" {
            # "Clear Last Error?"
            n80 = Unbundle By Name(w237) -> ("Core.Last Error.remaining states"=w239:string, "Core.Shutdown?"=w240:bool)
            n81 = Unbundle By Name(w237) -> ("Core.Last Error.error"=w243:errorcluster)
            n82 = case shown="False" FALSE {
              tunnel: w243 -> [w251 _]
              tunnel: [w251 _] -> w242
              frame False {
              }
              frame True {
              }
            }
            n83 = case shown="False" w240 {
              tunnel: w239 -> [w248 w250]
              tunnel: [w248 w249] -> w236
              frame False {
                # "These are the remaining states (at the moment the error occured). States can be altered according to business logic."
                # "NOT SHUTTING DOWN"
              }
              frame True {
                # "Developer can decide to alter the states but should be aware that during the shutdown process, there are certain states that must be run for the SMO to properly shut itself (and this process) down. As such, one can add states to perform additional clean-ups, but should append the remaining state to be executed."
                # "SHUTTING DOWN"
                n84 = call <vilib>:"Add State(s) to Queue__jki_lib_state_machine.vi"("State(s) in (\"\")"=w250) -> ("States Out"=w249:string)  [unwired: 14 in]
              }
            }
            n85 = Bundle By Name(cluster=w237, "Core.Last Error.error"=w242) -> (w238:T5)
            n86 = call <vilib>:"Add State(s) to Queue__jki_lib_state_machine.vi"("State(s) in Front (\"\")"=w236, "State(s) in (\"\")"=w247) -> ("States Out"=w246:string)  [unwired: 13 in]
          }
          frame "Macro: Run Sequence" {
            # "0,1,2,3,4,"
            # "5"
            # "Do not put any code in this frame.\n(It is a separator no-op. You can make a copy of this frame to create a new Macro frame)"
            n87 = Unbundle By Name(w258) -> ("sequence"=w254:string[], "Running Step"=w252:i32)
            n88 = Array Size(array=w254) -> (size(s)=w264:i32)
            n89 = Index Array(array=w254, index=w252) -> (element=w253:string)
            n90 = Greater Or Equal?(x=w264, y=w252) -> (x >= y?=w256:bool)
            n91 = Select(t=-1 ("Running Step"), s=w256, f=w252) -> (s? t:f=w263:i32)
            n92 = Bundle By Name(cluster=w258, "Running Step"=w263) -> (w259:T5)
            n93 = Select(t="Sequence: Status >> ...", s=w256, f="Idle //Check Event Structure\nMacro: Run Sequence" ("State(s) at Back (\"\")")) -> (s? t:f=w255:string)
            n94 = call <vilib>:"Add State(s) to Queue__jki_lib_state_machine.vi"("State(s) in Front (\"\")"=w253, "State(s) at Back (\"\")"=w255) -> ("States Out"=w257:string)  [unwired: 13 in]
            n95 = call <vilib>:"Add State(s) to Queue__jki_lib_state_machine.vi"("State(s) in Front (\"\")"=w257, "State(s) in (\"\")"=w268) -> ("States Out"=w267:string)  [unwired: 13 in]
          }
          frame "Macro: Debug" {
            # "exe?"
            # "If pane is an EXE, then close it when we exit"
            # "Macro: Debug\n(get debug behavior, determine UI and determine shutdown behavior)"
            n96 = Unbundle By Name(w272) -> ("Core.Close Panel on Exit?"=w275:bool, "SelfRef"=w280:refnum<class "Instrument.AFM_DLog.lvclass">)
            n97 = property class="App"() -> ("App.Kind"=w278:T1)  [unwired: 2 in, 2 out]
            n98 = Equal?(x=w278, y=T1."Run Time System" ("Application:Kind")) -> (x = y?=w274:bool)
            n99 = call <userlib>:"Get Debug Mode.vi"("error in (no error)"=w270, "SMO"=w280) -> ("error out"=w271:errorcluster, "Behavior"=w279:T7)  [unwired: 7 in, 1 out]
            n100 = case shown="\"Normal\", Default" w279 {
              tunnel: [w284 w286] -> w276
              tunnel: w275 -> [w284 _]
              tunnel: w274 -> [_ w288]
              tunnel: [_ "UI: Front Panel State >> Open\nUI: Wait >> 1000"] -> w269
              frame "Normal", Default {
                # "respect core.close"
              }
              frame "Debug" {
                # "keep panel open\nunless exe"
                n101 = Or(x=w288, y=FALSE) -> (x .or. y?=w286:bool)
              }
            }
            n102 = Bundle By Name(cluster=w272, "Core.Close Panel on Exit?"=w276) -> (w273:T5)
            n103 = call <vilib>:"Add State(s) to Queue__jki_lib_state_machine.vi"("State(s) in Front (\"\")"=w269, "State(s) in (\"\")"=w283) -> ("States Out"=w282:string)  [unwired: 13 in]
          }
          frame "Macro: Exit" {
            # "Exit Macro\n(This is called once, when the VI exits)"
            n104 = Unbundle By Name(w290) -> ("Core.Close Panel on Exit?"=w303:bool)
            n105 = Select(t="UI: Front Panel State >> Close", s=w303, f="" ("Empty String Constant")) -> (s? t:f=w301:string)
            n106 = Bundle By Name(cluster=w290, "Core.Shutdown?"=TRUE) -> (w291:T5)
            n107 = call <vilib>:"Add State(s) to Queue__jki_lib_state_machine.vi"("State(s) in Front (\"\")"="Data: Cleanup\nEvents: Unregister", "State(s) in (\"\")"="Process: Sync", "State(s) at Back (\"\")"="Exit") -> ("States Out"=w296:string)  [unwired: 12 in]
            n108 = call <vilib>:"Add State(s) to Queue__jki_lib_state_machine.vi"("State(s) in Front (\"\")"="Instrument: Close", "State(s) in (\"\")"=w301, "State(s) at Back (\"\")"=w296) -> ("States Out"=w300:string)  [unwired: 12 in]
            n109 = call <vilib>:"Add State(s) to Queue__jki_lib_state_machine.vi"("State(s) in Front (\"\")"=w300, "State(s) in (\"\")"=w305) -> ("States Out"=w304:string)  [unwired: 13 in]
          }
          frame "---------- Process ----------" {
            # "Template Separator\n(You can make a copy of, or modify, this frame)"
            n110 = call <vilib>:"Add State(s) to Queue__jki_lib_state_machine.vi"("State(s) in (\"\")"=w310) -> ("States Out"=w309:string)  [unwired: 14 in]
          }
          frame "Process: Sync" {
            n111 = Unbundle By Name(w318) -> ("SelfRef"=w314:refnum<class "Instrument.AFM_DLog.lvclass">)
            n112 = call <vilib>:"WaitOnProcessSync.vi"("error in (no error)"=w313, "SMO"=w314) -> ("error out"=w312:errorcluster, "Don't run?"=w317:bool)  [unwired: 7 in, 1 out]
            n113 = Select(t="Data: Cleanup\nEvents: Unregister\nExit", s=w317, f="" ("Empty String Constant")) -> (s? t:f=w311:string)
            n114 = call <vilib>:"Add State(s) to Queue__jki_lib_state_machine.vi"("State(s) in Front (\"\")"=w311, "State(s) in (\"\")"=w321) -> ("States Out"=w320:string)  [unwired: 13 in]
          }
          frame "---------- Events ----------" {
            # "Template Separator\n(You can make a copy of, or modify, this frame)"
            n115 = call <vilib>:"Add State(s) to Queue__jki_lib_state_machine.vi"("State(s) in (\"\")"=w326) -> ("States Out"=w325:string)  [unwired: 14 in]
          }
          frame "Events: Register" {
            n116 = Unbundle By Name(w332) -> ("SelfRef"=w333:refnum<class "Instrument.AFM_DLog.lvclass">)
            n117 = call <vilib>:"GetProtectedEvents.vi"("SMO"=w333) -> ("error out"=w331:errorcluster, "SMO Protected Events"=w336:T8, "SMO out"=w330:refnum<class "Instrument.AFM_DLog.lvclass">)  [unwired: 8 in]
            n118 = call "Instrument-Template.GetPrivateEvents.vi"("Instrument.AFM_DLog in"=w330) -> ("error out"=w327:errorcluster, "AFM_DLog Private Events"=w328:cluster{"MessageToProcess":refnum<user-event>})  [unwired: 8 in, 1 out]
            n119 = register-events(w336, w328) -> (reference out=w337:refnum<event-registration>, error out=w334:errorcluster)  [unwired: 2 in]
            n120 = Merge Errors(w334, w327, w331, w329) -> (w335:errorcluster)
            n121 = call <vilib>:"Add State(s) to Queue__jki_lib_state_machine.vi"("State(s) in (\"\")"=w339) -> ("States Out"=w338:string)  [unwired: 14 in]
          }
          frame "Events: Unregister" {
            n122 = Unregister For Events(event registration refnum=w342, error in=w341) -> (error out=w340:errorcluster)
            n123 = call <vilib>:"Clear Errors.vi"("error in (no error)"=w340) -> ()  [unwired: 5 in, 2 out]
            n124 = call <vilib>:"Add State(s) to Queue__jki_lib_state_machine.vi"("State(s) in (\"\")"=w345) -> ("States Out"=w344:string)  [unwired: 14 in]
          }
          frame "---------- Instrument ----------" {
            n125 = Unbundle By Name(w348) -> ("SelfRef"=w346:refnum<class "Instrument.AFM_DLog.lvclass">, "HAL"=w347:refnum<class "HAL.lvclass">)
            n126 = Bundle By Name(cluster=w348, "SelfRef"=w346, "HAL"=w347) -> (w349:T5)
            n127 = call <vilib>:"Add State(s) to Queue__jki_lib_state_machine.vi"("State(s) in (\"\")"=w353) -> ("States Out"=w352:string)  [unwired: 14 in]
          }
          frame "Instrument: Open" {
            n128 = Unbundle By Name(w358) -> ("SelfRef"=w356:refnum<class "Instrument.AFM_DLog.lvclass">)
            n129 = call-dynamic "Open Hardware.vi"("error in (no error)"=w357, "Instrument in"=w356) -> ("error out"=w354:errorcluster, "Instrument out"=w355:refnum<class "Instrument.AFM_DLog.lvclass">)  [unwired: 8 in]
            n130 = Bundle By Name(cluster=w358, "SelfRef"=w355) -> (w359:T5)
            n131 = call <vilib>:"Add State(s) to Queue__jki_lib_state_machine.vi"("State(s) in (\"\")"=w362) -> ("States Out"=w361:string)  [unwired: 14 in]
          }
          frame "Instrument: Write" {
            n132 = Unbundle By Name(w367) -> ("SelfRef"=w364:refnum<class "Instrument.AFM_DLog.lvclass">)
            n133 = call-dynamic "Write Hardware.vi"("error in (no error)"=w365, "Instrument in"=w364) -> ("error out"=w366:errorcluster, "Instrument out"=w363:refnum<class "Instrument.AFM_DLog.lvclass">)  [unwired: 8 in]
            n134 = Bundle By Name(cluster=w367, "SelfRef"=w363) -> (w368:T5)
            n135 = call <vilib>:"Add State(s) to Queue__jki_lib_state_machine.vi"("State(s) in (\"\")"=w371) -> ("States Out"=w370:string)  [unwired: 14 in]
          }
          frame "Instrument: Read" {
            n136 = Unbundle By Name(w377) -> ("SelfRef"=w373:refnum<class "Instrument.AFM_DLog.lvclass">)
            n137 = call-dynamic "Read Hardware.vi"("error in (no error)"=w375, "Instrument in"=w373) -> ("error out"=w376:errorcluster, "response"=w374:string, "Instrument out"=w372:refnum<class "Instrument.AFM_DLog.lvclass">)  [unwired: 7 in]
            n138 = Bundle By Name(cluster=w377, "SelfRef"=w372, "MessageToProcess.Message.Data"=w374) -> (w378:T5)
            n139 = call <vilib>:"Add State(s) to Queue__jki_lib_state_machine.vi"("State(s) in (\"\")"=w381) -> ("States Out"=w380:string)  [unwired: 14 in]
          }
          frame "Instrument: Close" {
            n140 = Unbundle By Name(w386) -> ("SelfRef"=w383:refnum<class "Instrument.AFM_DLog.lvclass">)
            n141 = call-dynamic "Close Hardware.vi"("error in (no error)"=w384, "Instrument in"=w383) -> ("error out"=w385:errorcluster, "Instrument out"=w382:refnum<class "Instrument.AFM_DLog.lvclass">)  [unwired: 8 in]
            n142 = Bundle By Name(cluster=w386, "SelfRef"=w382) -> (w387:T5)
            n143 = call <vilib>:"Add State(s) to Queue__jki_lib_state_machine.vi"("State(s) in (\"\")"=w390) -> ("States Out"=w389:string)  [unwired: 14 in]
          }
          frame "Instrument: Do Something" {
            # "communicate with\nhardware"
            n144 = Unbundle By Name(w401) -> ("SelfRef"=w400:refnum<class "Instrument.AFM_DLog.lvclass">, "MessageToProcess.Message.Data"=w398:variant, "MessageToProcess.Message.ID"=w393:string)
            n145 = call "Instrument-Template.doSomethingExample.vi"("error in (no error)"=w399, "Data"=w398, "Instrument.AFM_DLog in"=w400) -> ("error out"=w394:errorcluster, "Data out"=w392:variant, "Instrument.AFM_DLog out"=w397:refnum<class "Instrument.AFM_DLog.lvclass">)  [unwired: 6 in]
            n146 = Empty String/Path?(string/path=w392) -> (empty?=w391:bool)
            n147 = case shown="False" w391 {
              tunnel: w397 -> [w410 w412]
              tunnel: [w407 w412] -> w396
              tunnel: [w406 w411] -> w395
              tunnel: w392 -> [w409 _]
              tunnel: w394 -> [w408 w411]
              tunnel: w393 -> [_ _]
              frame False {
                # "send data to\ninstrument:process.vi"
                n148 = call <userlib>:"setAllData.vi"("error in (no error)"=w408, "AllData"=w409, "Instrument in"=w410) -> ("error out"=w406:errorcluster, "Instrument out"=w407:refnum<class "Instrument.AFM_DLog.lvclass">)  [unwired: 7 in]
              }
              frame True {
              }
            }
            n149 = Bundle By Name(cluster=w401, "SelfRef"=w396) -> (w402:T5)
            n150 = call <vilib>:"Add State(s) to Queue__jki_lib_state_machine.vi"("State(s) in (\"\")"=w405) -> ("States Out"=w404:string)  [unwired: 14 in]
          }
          frame "Instrument: Log" {
            # "THIS process.vi is responsible for logging data. Logging can be triggered in the timeout (as shown in this template proces.vi's tieout case) OR it could be triggered by data changes, or any other way you can device.\n\nThe code above will log ALL data. But you have the ability to log a subset, log some items on a different schedule, etc."
            n151 = Unbundle By Name(w420) -> ("SelfRef"=w417:refnum<class "Instrument.AFM_DLog.lvclass">)  [unwired: 2 out]
            n152 = call-dynamic "Get SMO Database Paths.vi"("error in (no error)"=w416, "Instrument.AFM_DLog in"=w417) -> ("error out"=w414:errorcluster, "Paths"=w415:string, "Instrument.AFM_DLog out"=w413:refnum<class "Instrument.AFM_DLog.lvclass">)  [unwired: 7 in]
            n153 = call <userlib>:"Instrument.logToDatabase.vi"("error in (no error)"=w414, "Paths"=w415, "Instrument"=w413) -> ("error out"=w418:errorcluster, "Instrument out"=w419:refnum<class "Instrument.AFM_DLog.lvclass">)  [unwired: 7 in]
            n154 = Bundle By Name(cluster=w420, "SelfRef"=w419) -> (w421:T5)
            n155 = call <vilib>:"Add State(s) to Queue__jki_lib_state_machine.vi"("State(s) in (\"\")"=w424) -> ("States Out"=w423:string)  [unwired: 14 in]
          }
          frame "---------- Sequence ----------" {
            n156 = call <vilib>:"Add State(s) to Queue__jki_lib_state_machine.vi"("State(s) in (\"\")"=w429) -> ("States Out"=w428:string)  [unwired: 14 in]
          }
          frame "Sequence: Status" {
            # "Sequence: Status\n(Use this frame to pass the status to the UI, this VI's UI, etc)"
            n157 = call <vilib>:"Add State(s) to Queue__jki_lib_state_machine.vi"("State(s) in (\"\")"=w435) -> ("States Out"=w434:string)  [unwired: 14 in]
            "Status" <- w430
          }
          frame "Sequence: Wait" {
            # "Sequence: Wait\n(Non-Blocking Wait)"
            # "F = repeat this state. wait\nT = go to next state. don't wait"
            n158 = Unbundle By Name(w444) -> ("Running Step"=w437:i32)
            n159 = call <userlib>:"Wait Logic.vi"("error in (no error)"=w440, "Time"=w438) -> ("error out"=w439:errorcluster, "Status String"=w436:string, "Trigger"=w441:bool)  [unwired: 6 in, 1 out]
            n160 = Increment(x=w437) -> (x+1=w451:i32)
            n161 = Select(t=w451, s=w441, f=w437) -> (s? t:f=w442:i32)
            n162 = Select(t=u32 0, s=w441, f=u32 100 ("milliseconds to wait")) -> (s? t:f=w448:u32)
            n163 = call <userlib>:"Wait (ms)__ogtk.vi"("error in (no error)"=w439, "milliseconds to wait"=w448) -> ("error out"=w446:errorcluster)  [unwired: 8 in, 1 out]
            n164 = Bundle By Name(cluster=w444, "Running Step"=w442) -> (w443:T5)
            n165 = call <vilib>:"Build State String with Arguments__JKI_lib_State_Machine.vi"("Arguments (\"\")"=w436, "State"="Sequence: Status") -> ("State with Arguments"=w445:string)  [unwired: 4 in]
            n166 = call <vilib>:"Add State(s) to Queue__jki_lib_state_machine.vi"("State(s) in Front (\"\")"=w445, "State(s) in (\"\")"=w454) -> ("States Out"=w453:string)  [unwired: 13 in]
          }
        }
      }
    }
    frame Error {
    }
  }
  n167 = call-parent "Process.vi"("error in"=w5, "Instrument"=w4) -> ("error out"=w2:errorcluster, "Instrument out"=→"Instrument.AFM_DLog out":refnum<class "Instrument.AFM_DLog.lvclass">)  [unwired: 8 in]
  n168 = Merge Errors(w2, w1) -> (→"error out":errorcluster)
